vi "CSV_Image_Data_Append.vi"(0 "input cluster":T2={"L16 Linear Actuator"="", "XE 1000 Pump"="", "Camera1"="", "Camera2"="", "Img_Capt"=FALSE, "Actuator"=FALSE, "Pump"=FALSE, "Cam 1"=FALSE, "Cam 2"=FALSE, "Empty_Refill"=FALSE, "Crop"=FALSE, "Light intensity"=100, "Exposure Time"=1000.0, "Sample Name"="Test Sample", "Operator"="MRJ", "Calibration 1"=path "C:/Users/au540322/Desktop/IHS_Project/images/Debris/Debris_0/Debris_0_2019_06_01-23-32-49-686.PNG", "Calibration 2"=path "C:/Users/au540322/Desktop/IHS_Project/images/Debris/Debris_0/Debris_0_2019_06_01-23-32-49-686.PNG", "Framerate"=1, "Timeout Sample"=50, "Collection date"="MRJ", "Sample size threshold"=1, "Empty start"=1, "Command"="MRJ", "Station"="", "Species Name"="", "Other Notes"="", "Aperture"=enum."Item 0", "Image Process Queue Size"=10, "Image Save Queue Size"=1, "Overload threshold"=500, "Max Framerate"=100, "Rectangle 1"={"Left"=0, "Top"=0, "Right"=0, "Bottom"=0, "Rotation"=0.0}, "Rectangle 2"={"Left"=0, "Top"=0, "Right"=0, "Bottom"=0, "Rotation"=0.0}, "Detection Region %"=0.0, "Detect 1"=path "C:/Users/au540322/Desktop/IHS_Project/images/Debris/Debris_0/Debris_0_2019_06_01-23-32-49-686.PNG", "Detect 2"=path "C:/Users/au540322/Desktop/IHS_Project/images/Debris/Debris_0/Debris_0_2019_06_01-23-32-49-686.PNG", "Max large object threshold"=0, "Open(T)/Close(F)"=FALSE, "Img_Capt Begin"=FALSE, "Dispense Speed"=100, "Flush Size"=100, "Location"="Station", "Latitude"="Station", "Longitude"="Station", "Determiner"="Station", "Sex"="Station", "Camera1_Img"=refnum, "Camera2_Img"=refnum, "Img1_Orig_Disp"=refnum, "Img2_Orig_Disp"=refnum, "Img1_Orig_RGB"=refnum, "Img2_Orig_RGB"=refnum, "Blue_Plane_Extract"=refnum, "Subtracted_Plane"=refnum, "Img1_Binary"=refnum, "Img2_Binary"=refnum, "Crop_Mask"=refnum, "Img1_Save"=refnum, "Img2_Save"=refnum, "Img1_Cali_Full"=refnum, "Img2_Cali_Full"=refnum, "Img1_Cali_Detect"=refnum, "Img2_Cali_Detect"=refnum, "Cam 1 queue"=refnum, "Cam 2 queue"=refnum, "Cam 1 - save queue"=refnum, "Cam 2 - save queue"=refnum, "Overlay_Ring"=0, "SystemVersion"=0, "System Serial"="", "Legacy Cam Attributes"=FALSE} {"SystemVersion" items=["Standard", "XL"]; "Overlay_Ring" items=["Session Data", "Extended Setup", "Buffer", "Camera", "Dispenser", "Stats", "Connections"]; "Flush Size" min=1; "Dispense Speed" min=1; "Rectangle 2"."Rotation" format="%.2f"; "Rectangle 2"."Left" scale=0.0..1024.0; "Rectangle 2"."Right" scale=0.0..1024.0; "Rectangle 1"."Rotation" format="%.2f"; "Rectangle 1"."Left" scale=0.0..1024.0; "Rectangle 1"."Right" scale=0.0..1024.0; "Max Framerate" min=1; "Overload threshold" min=1; "Image Save Queue Size" min=1; "Image Process Queue Size" min=1; "Empty start" min=1; "Sample size threshold" min=1; "Framerate" min=1; "Light intensity" scale=0.0..100.0}, 1 "Image path":string, 2 "Sample Name":string, 3 "Image Name":string, 4 "Sample Data":dbl[](array[numeric]), 5 "ROI Descriptor":T1) -> ()   [LabVIEW 2022 SP3]
uses:
  controls/Data.ctl
  <vilib>/userdefined/High Color/IMAQdx.ctl
  <vilib>/vision/Image Controls.llb/IMAQ Image.ctl
  <vilib>/Utility/file.llb/Write Delimited Spreadsheet (string).vi
panel:
  out "string":string
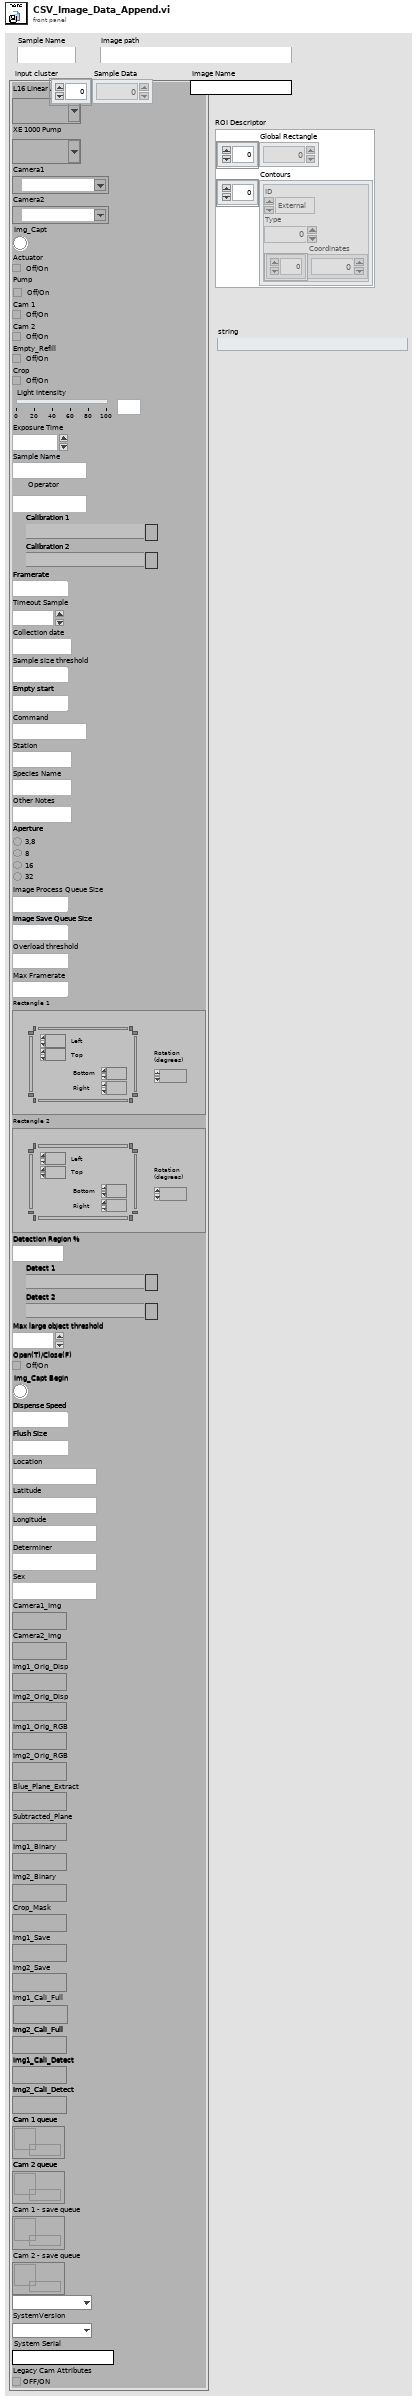
[diagram p1: front panel]
types:
  T1 = cluster{"Global Rectangle":i32[], "Contours":cluster{"ID":enum32{"External", "Internal"}, "Type":u32, "Coordinates":i32[]}[]}
  T2 = typedef "Data.ctl" = cluster{"L16 Linear Actuator":refnum<visa-resource-name>, "XE 1000 Pump":refnum<visa-resource-name>, "Camera1":T3, "Camera2":T3, "Img_Capt":bool, "Actuator":bool, "Pump":bool, "Cam 1":bool, "Cam 2":bool, "Empty_Refill":bool, "Crop":bool, "Light intensity":i32, "Exposure Time":dbl, "Sample Name":string, "Operator":string, "Calibration 1":path, "Calibration 2":path, "Framerate":i32, "Timeout Sample":i32, "Collection date":string, "Sample size threshold":i32, "Empty start":u32, "Command":string, "Station":string, "Species Name":string, "Other Notes":string, "Aperture":enum32{"Item 0", "Item 1", "Item 2", "Item 3"}, "Image Process Queue Size":i32, "Image Save Queue Size":i32, "Overload threshold":i32, "Max Framerate":i32, "Rectangle 1":T4, "Rectangle 2":T4, "Detection Region %":dbl, "Detect 1":path, "Detect 2":path, "Max large object threshold":i32, "Open(T)/Close(F)":bool, "Img_Capt Begin":bool, "Dispense Speed":i32, "Flush Size":i32, "Location":string, "Latitude":string, "Longitude":string, "Determiner":string, "Sex":string, "Camera1_Img":T5, "Camera2_Img":T5, "Img1_Orig_Disp":T5, "Img2_Orig_Disp":T5, "Img1_Orig_RGB":T5, "Img2_Orig_RGB":T5, "Blue_Plane_Extract":T5, "Subtracted_Plane":T5, "Img1_Binary":T5, "Img2_Binary":T5, "Crop_Mask":T5, "Img1_Save":T5, "Img2_Save":T5, "Img1_Cali_Full":T5, "Img2_Cali_Full":T5, "Img1_Cali_Detect":T5, "Img2_Cali_Detect":T5, "Cam 1 queue":refnum<queue>, "Cam 2 queue":refnum<queue>, "Cam 1 - save queue":refnum<queue>, "Cam 2 - save queue":refnum<queue>, "Overlay_Ring":u16, "SystemVersion":u16, "System Serial":string, "Legacy Cam Attributes":bool}
  T3 = typedef "IMAQdx.ctl" = refnum<k21>
  T4 = typedef "IMAQ Rectangle" = cluster{"Left":i32, "Top":i32, "Right":i32, "Bottom":i32, "Rotation":dbl}
  T5 = typedef "IMAQ Image.ctl" = refnum<image>
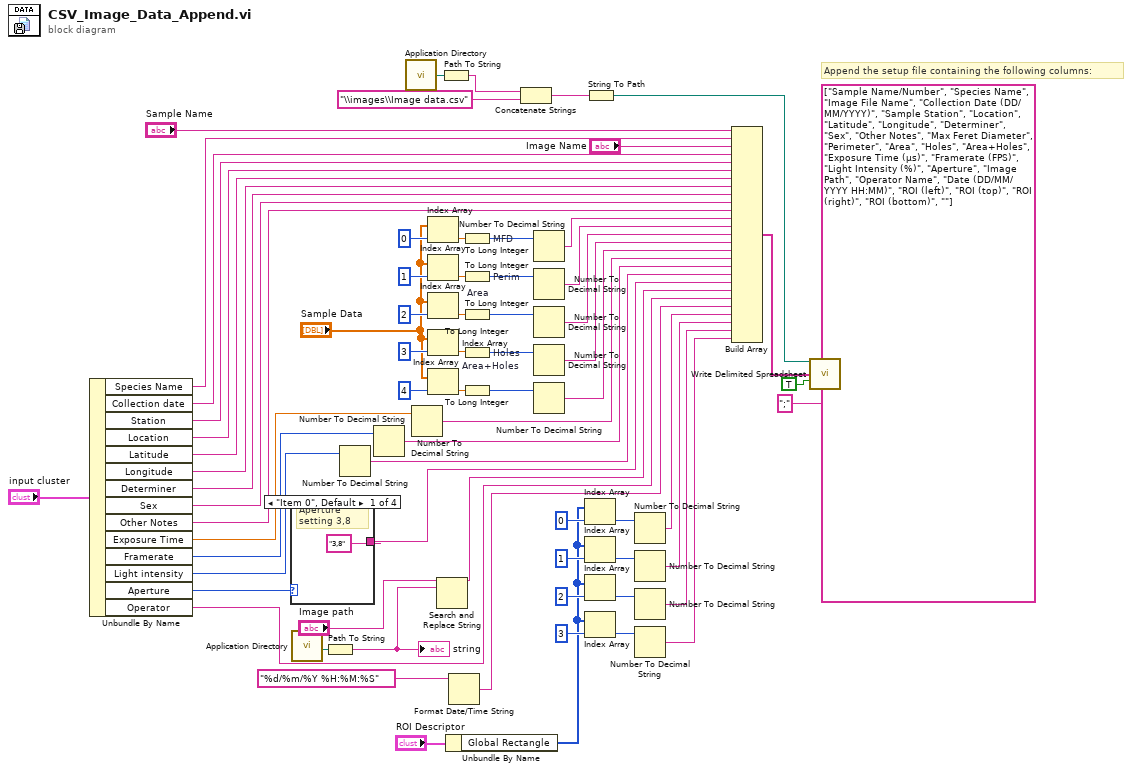
[diagram p0: block diagram]
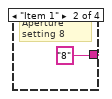
[diagram p2: hidden frame]
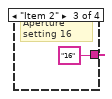
[diagram p3: hidden frame]
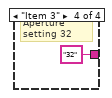
[diagram p4: hidden frame]
diagram:
  (unwired) string[] ["Sample Name/Number", "Species Name", "Image File Name", "Collection Date (DD/MM/YYYY)", "Sample Station", "Location", "Latitude", "Longitude", "Determiner", "Sex", "Other Notes", "Max Feret Diameter", "Perimeter", "Area", "Holes", "Area+Holes", "Exposure Time (µs)", "Framerate (FPS)", "Light Intensity (%)", "Aperture", "Image Path", "Operator Name", "Date (DD/MM/YYYY HH:MM)", "ROI (left)", "ROI (top)", "ROI (right)", "ROI (bottom)", ""]
  # "Append the setup file containing the following columns:"
  n1 = Unbundle By Name("input cluster") -> ("Species Name"=w41:string, "Collection date"=w42:string, "Station"=w43:string, "Location"=w44:string, "Latitude"=w45:string, "Longitude"=w46:string, "Determiner"=w47:string, "Sex"=w48:string, "Other Notes"=w49:string, "Exposure Time"=w59:dbl, "Framerate"=w1:i32, "Light intensity"=w58:i32, "Aperture"=w57:enum32{"Item 0", "Item 1", "Item 2", "Item 3"}, "Operator"=w51:string)
  n2 = case shown="\"Item 0\", Default" w57 {
    tunnel: ["3,8" "8" "16" "32"] -> w53
    frame "Item 0", Default {
      # "Aperture setting 3,8"
    }
    frame "Item 1" {
      # "Aperture setting 8"
    }
    frame "Item 2" {
      # "Aperture setting 16"
    }
    frame "Item 3" {
      # "Aperture setting 32"
    }
  }
  n3 = call <vilib>:"Application Directory.vi"() -> ("Application Directory"=w63:path)
  n4 = Path To String(path=w63) -> (string=w61:string)
  "string" <- w61
  n5 = Number To Decimal String(number=w58) -> (decimal integer string=w54:string)  [unwired: 1 in]
  n6 = Number To Decimal String(number=w1) -> (decimal integer string=w55:string)  [unwired: 1 in]
  n7 = call <vilib>:"Application Directory.vi"() -> ("Application Directory"=w67:path)
  n8 = Number To Decimal String(number=w59) -> (decimal integer string=w56:string)  [unwired: 1 in]
  n9 = Index Array ("MFD")(array="Sample Data", index=0) -> (element=w31:dbl)
  n10 = Index Array ("MFD")(array="Sample Data", index=1) -> (element=w26:dbl)
  n11 = Index Array ("MFD")(array="Sample Data", index=2) -> (element=w24:dbl)
  n12 = Index Array ("MFD")(array="Sample Data", index=3) -> (element=w25:dbl)
  n13 = Index Array ("MFD")(array="Sample Data", index=4) -> (element=w22:dbl)
  n14 = Search and Replace String(input string="Image path", search string=w61) -> (result string=w52:string)  [unwired: 6 in, 3 out]
  n15 = Path To String(path=w67) -> (string=w66:string)
  n16 = Unbundle By Name("ROI Descriptor") -> ("Global Rectangle"=w6:i32[])
  n17 = Format Date/Time String(time format string (%c)="%d/%m/%Y %H:%M:%S") -> (date/time string=w50:string)  [unwired: 2 in]
  n18 = To Long Integer "MFD"(number=w31) -> (32bit integer=w37:i32)
  n19 = To Long Integer "Perim"(number=w26) -> (32bit integer=w36:i32)
  n20 = To Long Integer "Area"(number=w24) -> (32bit integer=w35:i32)
  n21 = To Long Integer "Holes"(number=w25) -> (32bit integer=w34:i32)
  n22 = To Long Integer "Area+Holes"(number=w22) -> (32bit integer=w33:i32)
  n23 = Concatenate Strings(w66, "\\images\\Image data.csv") -> (w64:string)
  n24 = Number To Decimal String(number=w37) -> (decimal integer string=w21:string)  [unwired: 1 in]
  n25 = Number To Decimal String(number=w36) -> (decimal integer string=w20:string)  [unwired: 1 in]
  n26 = Number To Decimal String(number=w35) -> (decimal integer string=w19:string)  [unwired: 1 in]
  n27 = Number To Decimal String(number=w34) -> (decimal integer string=w18:string)  [unwired: 1 in]
  n28 = Number To Decimal String(number=w33) -> (decimal integer string=w17:string)  [unwired: 1 in]
  n29 = Index Array ("MFD")(array=w6, index=0) -> (element=w14:i32)
  n30 = Index Array ("MFD")(array=w6, index=1) -> (element=w13:i32)
  n31 = Index Array ("MFD")(array=w6, index=2) -> (element=w12:i32)
  n32 = Index Array ("MFD")(array=w6, index=3) -> (element=w11:i32)
  n33 = String To Path(string=w64) -> (path=w60:path)
  n34 = Number To Decimal String(number=w14) -> (decimal integer string=w5:string)  [unwired: 1 in]
  n35 = Number To Decimal String(number=w13) -> (decimal integer string=w4:string)  [unwired: 1 in]
  n36 = Number To Decimal String(number=w12) -> (decimal integer string=w3:string)  [unwired: 1 in]
  n37 = Number To Decimal String(number=w11) -> (decimal integer string=w2:string)  [unwired: 1 in]
  n38 = Build Array("Sample Name", w41, "Image Name", w42, w43, w44, w45, w46, w47, w48, w49, w21, w20, w19, w18, w17, w56, w55, w54, w53, w52, w51, w50, w5, w4, w3, w2) -> (w38:string[])
  n39 = call-poly <vilib>:"Write Delimited Spreadsheet.vi"("file path (dialog if empty)"=w60, "1D data"=w38, "append to file? (new file:F)"=TRUE, "delimiter (\\t)"=";" ("delimiter (\\t)")) -> ()  [unwired: 10 in, 2 out]
